vi "SIM BDF manager.vi"(1 "Simulation data":T1={"continuous integrator"=enum."RK 1 (Euler)", "initial time"=0.0, "final time"=6.0, "step size"=0.0, "proposed step size"=0.001, "max step size"=1e-06, "min step size"=0.0, "discrete time step"=0.0, "max step ratio"=3.0, "Diag Eval Stage"=enum."Major Substep", "Substep Index"=0, "Timestep Index"=10.0, "simulation time"=0.0, "current timestep base"=0.1, "proposed step time"=0.0, "absolute tolerance"=0.0, "relative tolerance"=0.0, "step accepted?"=FALSE, "step complete?"=FALSE, "Halt?"=FALSE, "reset integrator?"=FALSE, "machine epsilon"=1.0, "min float"=0.0, "error"={"status"=FALSE, "code"=0, "source"=""}, "Method Order"=0, "Finished Late [i-1]"=FALSE, "Discrete step?"=FALSE, "NaN and Inf check?"=FALSE, "Final Timestep Index"=0.0, "(maj+disc)or(init)?"=FALSE, "Full Solver Reset"=TRUE, "Execution Mode"=enum."Simulate to Completion", "check vector sizes?"=FALSE, "solver handles zc?"=FALSE, "Simulation Registry"={"Current Idx"=0, "Node Tags"=[], "Node Headers"=[], "Node Data"=[], "Cont State data"={"inputs"=[], "outputs"=[], "reset"=[], "lower limits"=[], "upper limits"=[], "limit types"=[], "reset types"=[], "initial conditions"=[], "reset I.C."=[], "limited?"=[], "State Names"=[]}, "DiscreteInfo"={"tick period (sec)"=0.0, "time (ticks)"=0, "fire?"=[], "registry"={"period (sec)"=[], "skew (sec)"=[], "period (tick)"=[], "skew (tick)"=[]}, "discrete \nblocks?"=FALSE, "steps per tick"=0.0, "steps to tick"=0.0, "discrete \ntick?"=FALSE}, "Disc State data"={"Disc States"=[], "State Names"=[]}, "Registry Error"={"Error Block ID"=0, "code"=0}, "ZC Indices"=[]}, "variable step solver?"=FALSE, "First Substep?"=FALSE, "Continuous States?"=FALSE} {"min float" format="%.1e"; "proposed step size" format="%.1e"; "proposed step time" format="%.1e"; "max step ratio" format="%.1e"; "min step size" format="%.1e"; "machine epsilon" format="%.1e"; "discrete time step" format="%.1e"; "max step size" format="%.1e"; "current timestep base" format="%.1e"; "final time" format="%.1e"; "simulation time" format="%.1e"; "relative tolerance" format="%.1e"; "absolute tolerance" format="%.1e"; "Substep Index" format="%.1e"; "step size" format="%.1e"; "initial time" format="%.1e"}) -> (0 "Simulation data out":T1={"continuous integrator"=enum."RK 1 (Euler)", "initial time"=0.0, "final time"=6.0, "step size"=0.0, "proposed step size"=0.001, "max step size"=1e-06, "min step size"=0.0, "discrete time step"=0.0, "max step ratio"=3.0, "Diag Eval Stage"=enum."Major Substep", "Substep Index"=0, "Timestep Index"=10.0, "simulation time"=0.0, "current timestep base"=0.1, "proposed step time"=0.0, "absolute tolerance"=0.0, "relative tolerance"=0.0, "step accepted?"=FALSE, "step complete?"=FALSE, "Halt?"=FALSE, "reset integrator?"=FALSE, "machine epsilon"=1.0, "min float"=0.0, "error"={"status"=FALSE, "code"=0, "source"=""}, "Method Order"=0, "Finished Late [i-1]"=FALSE, "Discrete step?"=FALSE, "NaN and Inf check?"=FALSE, "Final Timestep Index"=0.0, "(maj+disc)or(init)?"=FALSE, "Full Solver Reset"=TRUE, "Execution Mode"=enum."Simulate to Completion", "check vector sizes?"=FALSE, "solver handles zc?"=FALSE, "Simulation Registry"={"Current Idx"=0, "Node Tags"=[], "Node Headers"=[], "Node Data"=[], "Cont State data"={"inputs"=[], "outputs"=[], "reset"=[], "lower limits"=[], "upper limits"=[], "limit types"=[], "reset types"=[], "initial conditions"=[], "reset I.C."=[], "limited?"=[], "State Names"=[]}, "DiscreteInfo"={"tick period (sec)"=0.0, "time (ticks)"=0, "fire?"=[], "registry"={"period (sec)"=[], "skew (sec)"=[], "period (tick)"=[], "skew (tick)"=[]}, "discrete \nblocks?"=FALSE, "steps per tick"=0.0, "steps to tick"=0.0, "discrete \ntick?"=FALSE}, "Disc State data"={"Disc States"=[], "State Names"=[]}, "Registry Error"={"Error Block ID"=0, "code"=0}, "ZC Indices"=[]}, "variable step solver?"=FALSE, "First Substep?"=FALSE, "Continuous States?"=FALSE} {"min float" format="%.1e"; "proposed step size" format="%.1e"; "proposed step time" format="%.1e"; "max step ratio" format="%.1e"; "min step size" format="%.1e"; "machine epsilon" format="%.1e"; "discrete time step" format="%.1e"; "max step size" format="%.1e"; "current timestep base" format="%.1e"; "final time" format="%.1e"; "simulation time" format="%.1e"; "relative tolerance" format="%.1e"; "absolute tolerance" format="%.1e"; "Substep Index" format="%.1e"; "step size" format="%.1e"; "initial time" format="%.1e"})   [LabVIEW 2017]
uses:
  SIM simulation data.ctl
  SIM integration method.ctl
  SIM diagram eval stage.ctl
  SIMSCR Execution Mode.ctl
  SIM Simulation Registry.ctl
  SIM Registry Node Header.ctl
  SIM Registry Node Record.ctl
  SIM trigger type.ctl
  SIM solver state data.ctl
  SIM limit type.ctl
  SIM discrete data.ctl
  SIM Discrete state data.ctl
  SIM Simulation Registry Error.ctl
  SIM BDF stages.ctl
  SIM BDF data.ctl
  SIM Factored Matrix.ctl
panel:
  in  "Max Order":i32=5
  in  "max Newton iterations":i32=3
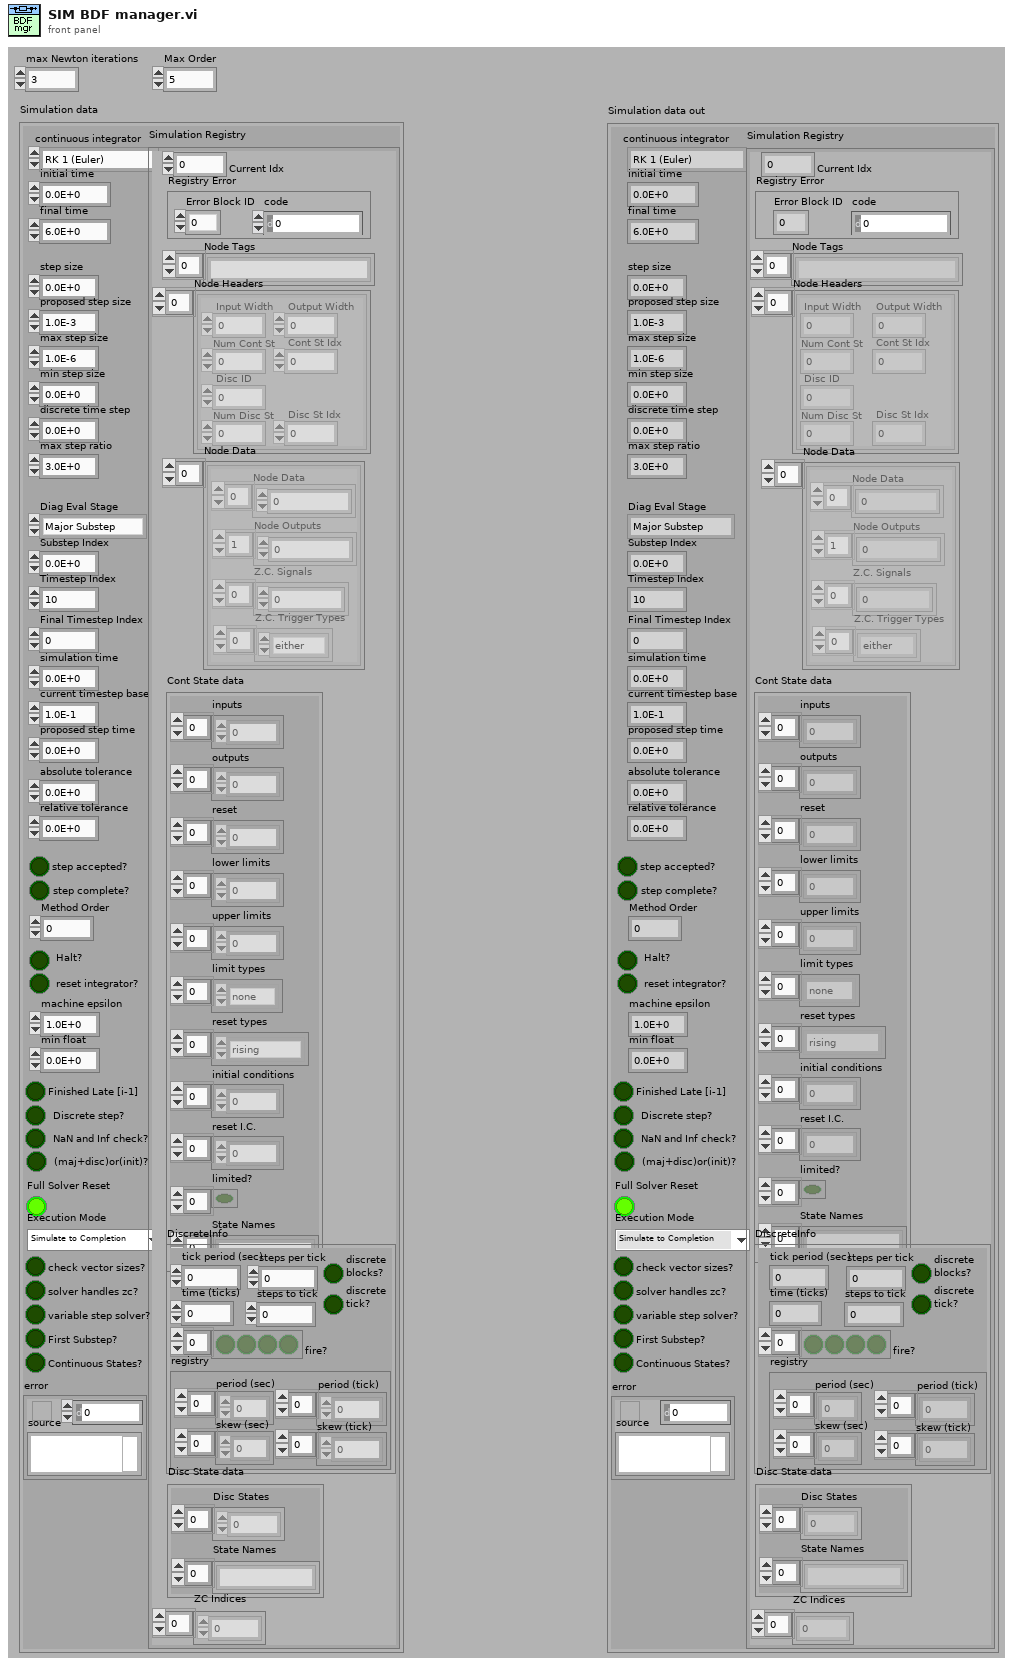
[diagram p1: front panel]
types:
  T1 = typedef "SIM simulation data.ctl" = cluster{"continuous integrator":T2, "initial time":dbl, "final time":dbl, "step size":dbl, "proposed step size":dbl, "max step size":dbl, "min step size":dbl, "discrete time step":dbl, "max step ratio":dbl, "Diag Eval Stage":T3, "Substep Index":i32, "Timestep Index":dbl, "simulation time":dbl, "current timestep base":dbl, "proposed step time":dbl, "absolute tolerance":dbl, "relative tolerance":dbl, "step accepted?":bool, "step complete?":bool, "Halt?":bool, "reset integrator?":bool, "machine epsilon":dbl, "min float":dbl, "error":errorcluster, "Method Order":u32, "Finished Late [i-1]":bool, "Discrete step?":bool, "NaN and Inf check?":bool, "Final Timestep Index":dbl, "(maj+disc)or(init)?":bool, "Full Solver Reset":bool, "Execution Mode":T4, "check vector sizes?":bool, "solver handles zc?":bool, "Simulation Registry":T5, "variable step solver?":bool, "First Substep?":bool, "Continuous States?":bool}
  T2 = typedef "SIM integration method.ctl" = enum16{"RK 1 (Euler)", "Linearizer", "State Query", "Trim Eval", "Adams", "RK 3", "RK 4", "RK 45", "BDF", "RK 2", "RK 23", "Rosenbrock", "Discrete States Only"}
  T3 = typedef "SIM diagram eval stage.ctl" = enum16{"Init", "Minor Substep", "Major Substep", "Final"}
  T4 = typedef "SIMSCR Execution Mode.ctl" = enum16{"Simulate to Completion", "Single Time-Step Simulation (Fixed Step Only)"}
  T5 = typedef "SIM Simulation Registry.ctl" = cluster{"Current Idx":i32, "Node Tags":string[], "Node Headers":T6[], "Node Data":T7[], "Cont State data":T9, "DiscreteInfo":T11, "Disc State data":T12, "Registry Error":T13, "ZC Indices":i32[]}
  T6 = typedef "SIM Registry Node Header.ctl" = cluster{"Input Width":i32, "Disc ID":i32, "Num Cont St":i32, "Cont St Idx":i32, "Num Disc St":i32, "Disc St Idx":i32, "Output Width":i32}
  T7 = typedef "SIM Registry Node Record.ctl" = cluster{"Node Data":dbl[], "Node Outputs":dbl[], "Z.C. Signals":dbl[], "Z.C. Trigger Types":T8[]}
  T8 = typedef "SIM trigger type.ctl" = enum16{"rising", "falling", "either", "none"}
  T9 = typedef "SIM solver state data.ctl" = cluster{"inputs":dbl[], "outputs":dbl[], "reset":dbl[], "lower limits":dbl[], "upper limits":dbl[], "limit types":T10[], "reset types":T8[], "initial conditions":dbl[], "reset I.C.":dbl[], "limited?":bool[], "State Names":string[]}
  T10 = typedef "SIM limit type.ctl" = enum16{"upper", "lower", "both", "none"}
  T11 = typedef "SIM discrete data.ctl" = cluster{"tick period (sec)":dbl, "time (ticks)":i32, "fire?":bool[], "registry":cluster{"period (sec)":dbl[], "skew (sec)":dbl[], "period (tick)":i32[], "skew (tick)":i32[]}, "discrete \nblocks?":bool, "steps per tick":dbl, "steps to tick":dbl, "discrete \ntick?":bool}
  T12 = typedef "SIM Discrete state data.ctl" = cluster{"Disc States":dbl[], "State Names":string[]}
  T13 = typedef "SIM Simulation Registry Error.ctl" = cluster{"Error Block ID":i32, "code":i32}
  T14 = typedef "SIM BDF stages.ctl" = enum16{"Init", "Initial Guess", "Compute Jacobian", "Newton Iteration", "Eval Error", "Choose StepSize", "Reset BDFs"}
  T15 = typedef "SIM BDF data.ctl" = cluster{"BDFs":dbl[][], "init. guess (y*)":dbl[], "p'(y*)":dbl[], "Factored jacobian":T16, "zero array":dbl[], "reinit Jac.":bool, "BDF stage":T14, "steps this jac":i32, "time index this jac":i32, "Number of jac evals":i32, "del_k":dbl[], "Current Order":i32, "Max Order":i32, "Steps This Order":i32, "Max Err Order":i32}
  T16 = typedef "SIM Factored Matrix.ctl" = cluster{"L":dbl[][], "U":dbl[][], "P":i32[][]}
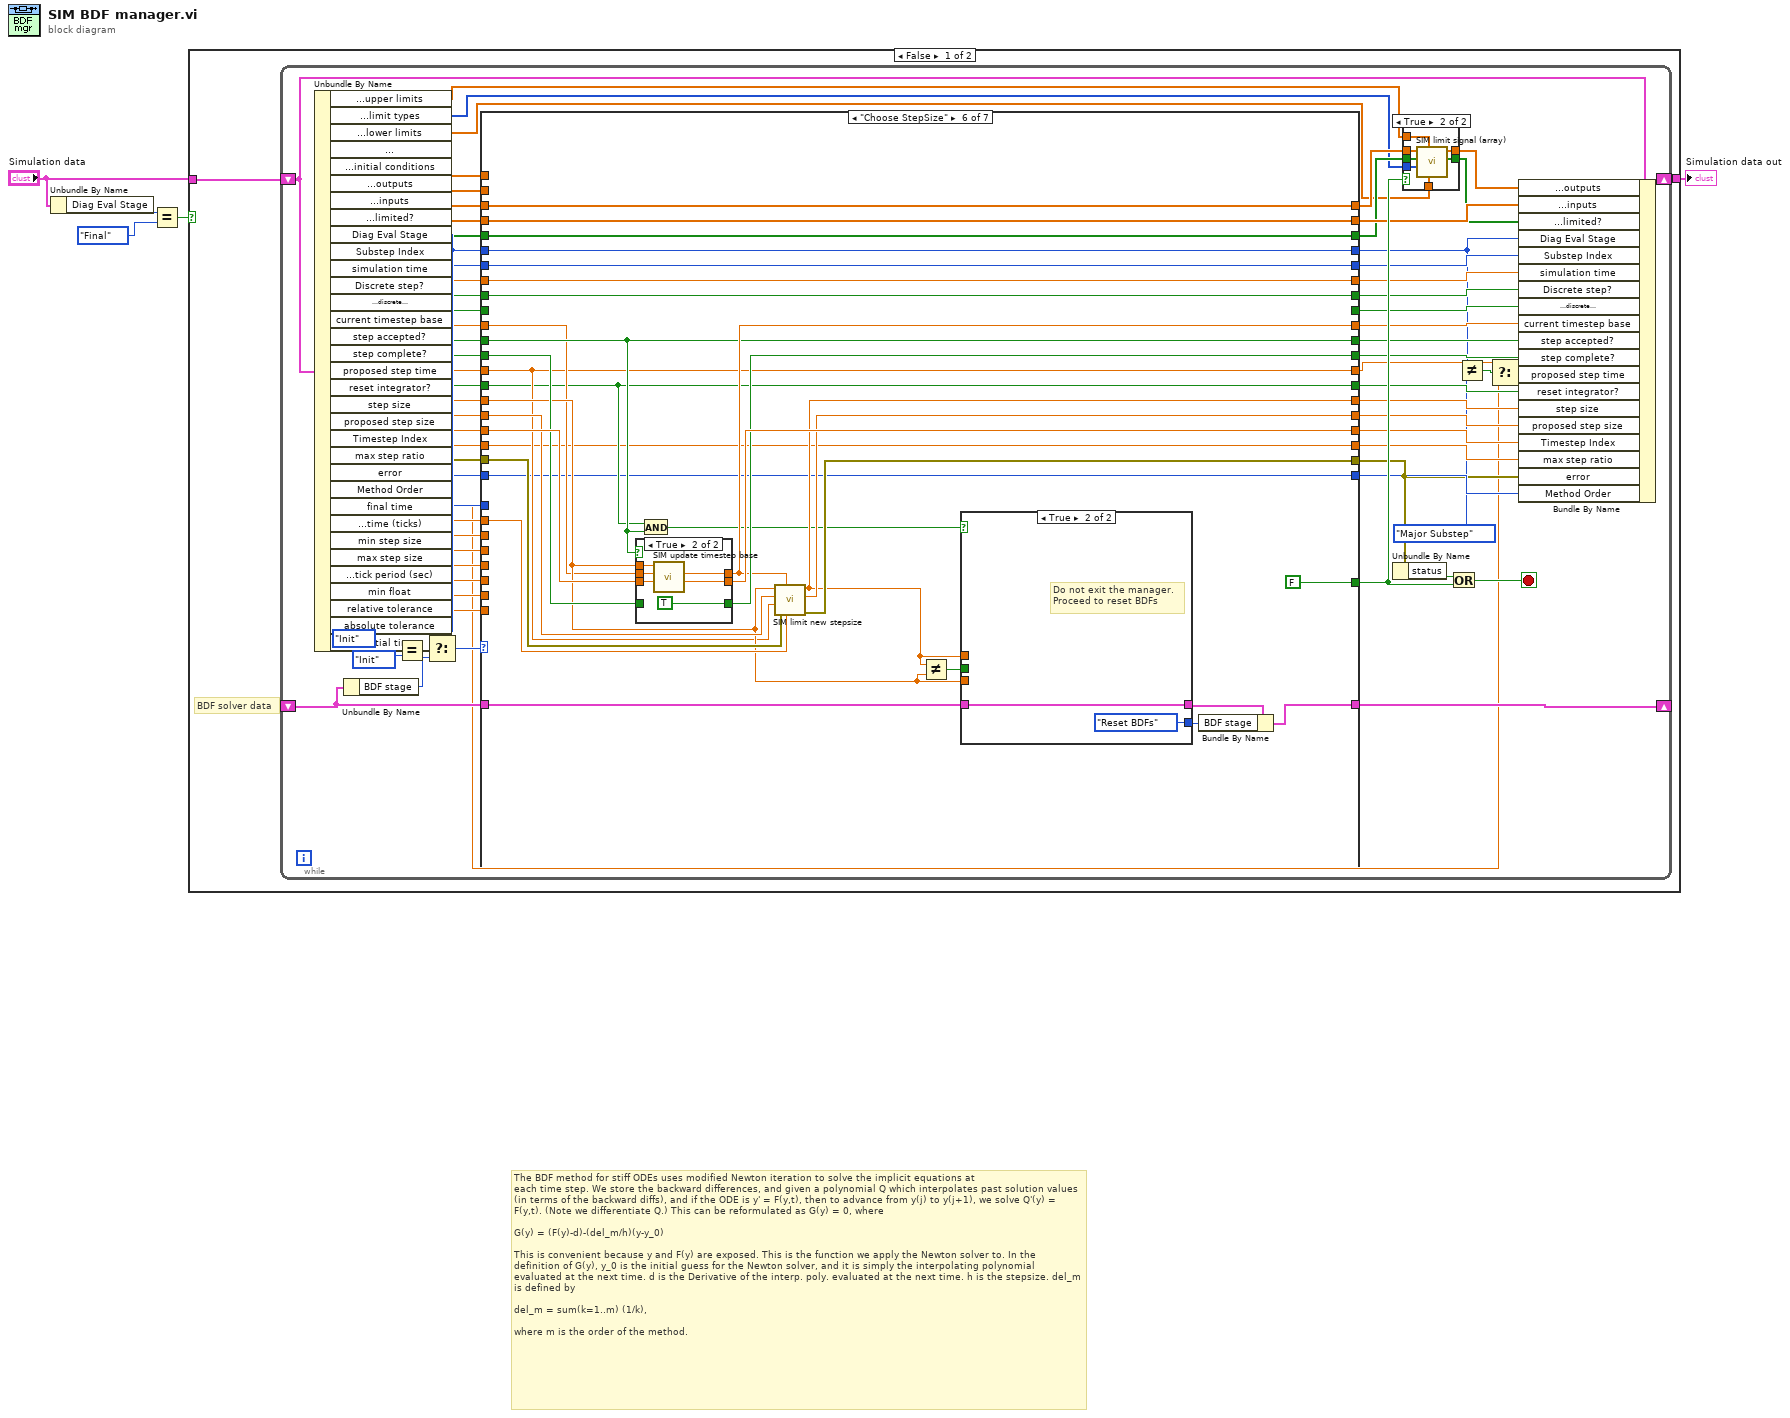
[diagram p0: block diagram]
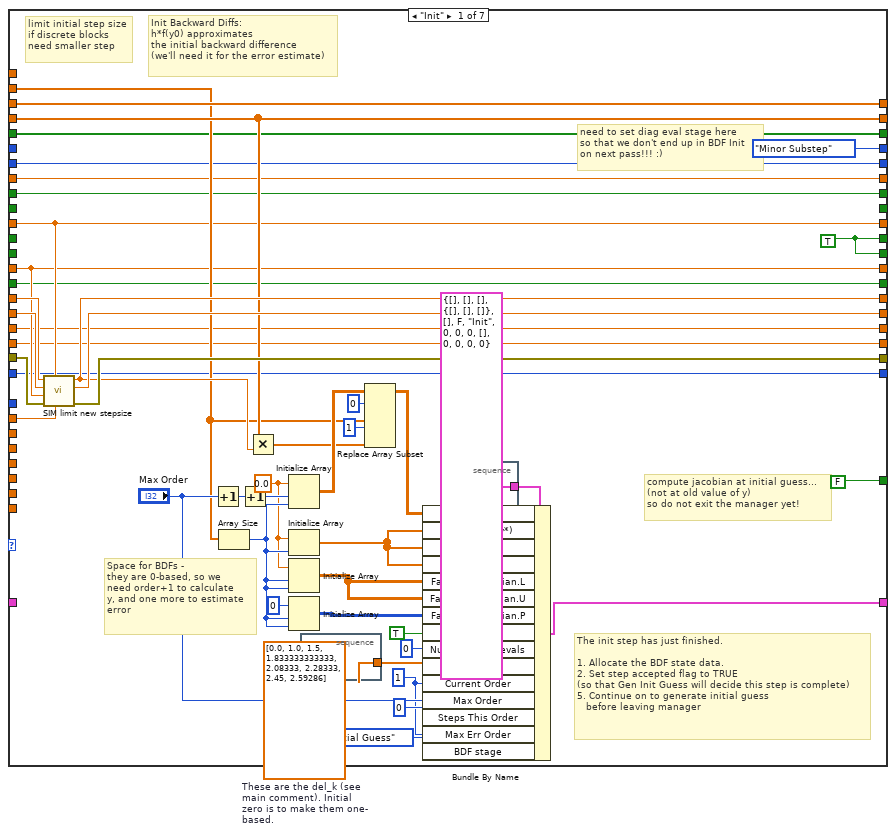
[diagram p3: hidden frame]
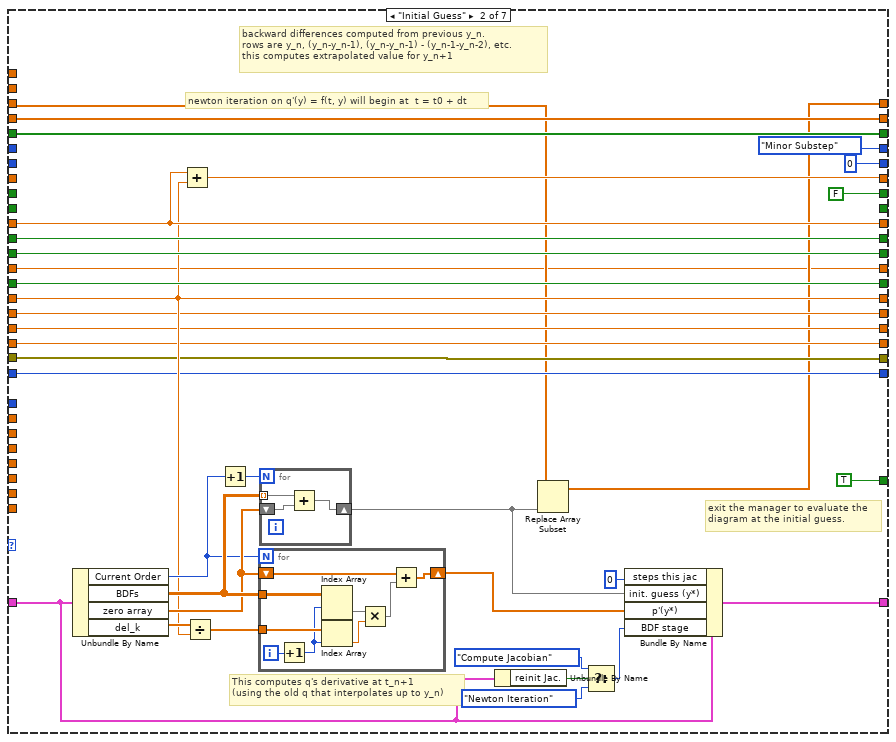
[diagram p4: hidden frame]
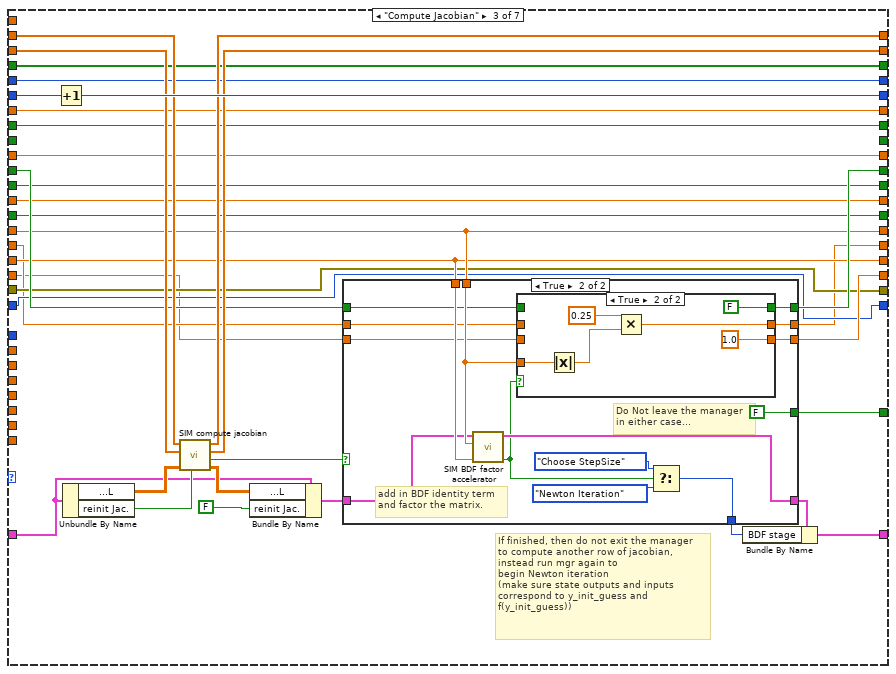
[diagram p5: hidden frame]
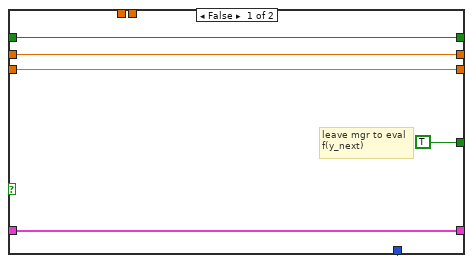
[diagram p6: hidden frame]
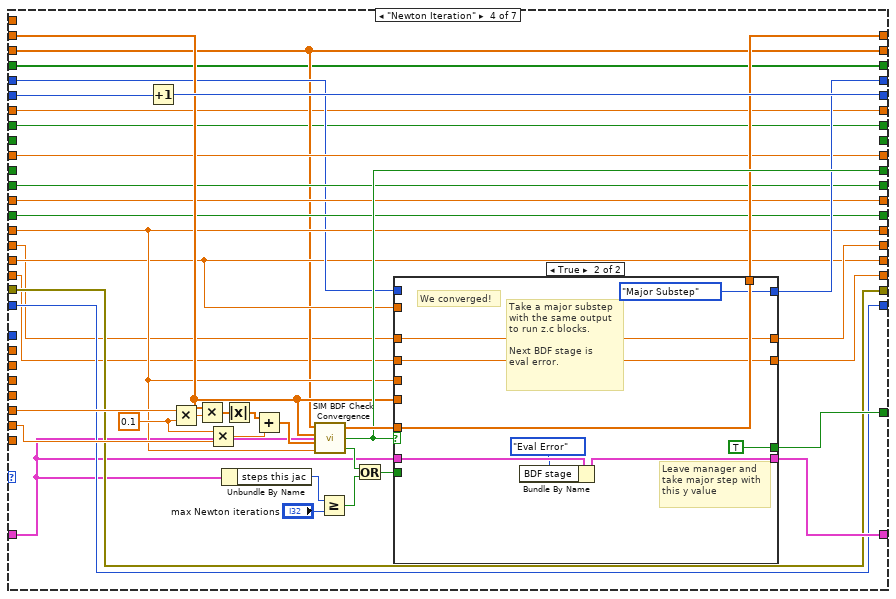
[diagram p8: hidden frame]
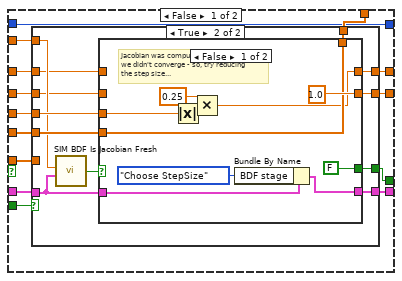
[diagram p9: hidden frame]
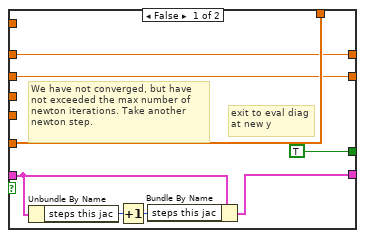
[diagram p10: hidden frame]
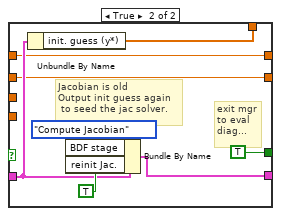
[diagram p11: hidden frame]
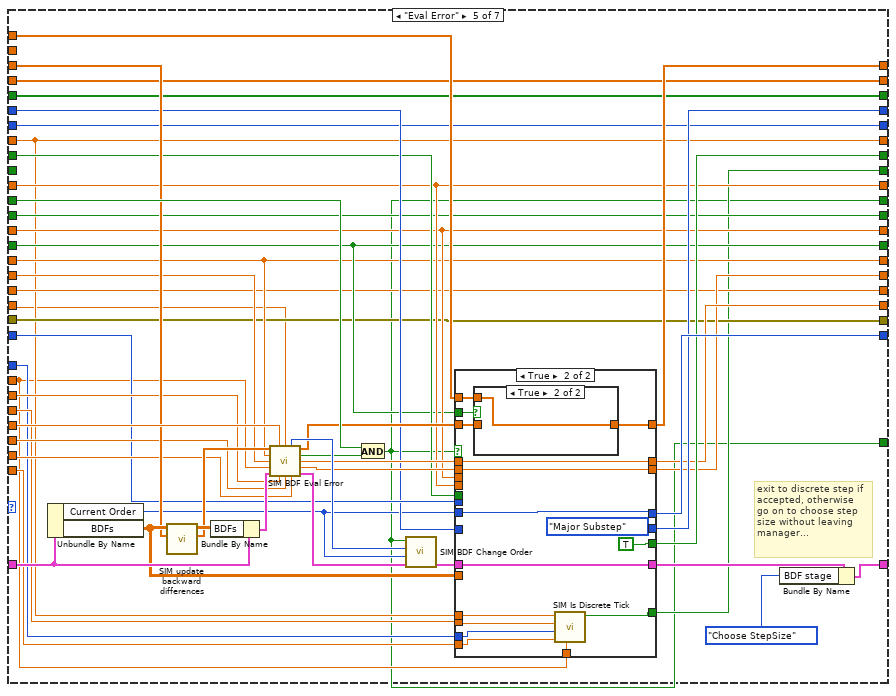
[diagram p12: hidden frame]
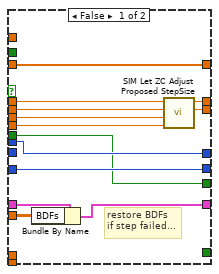
[diagram p13: hidden frame]
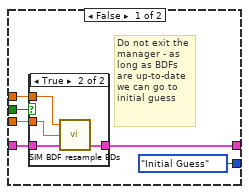
[diagram p15: hidden frame]
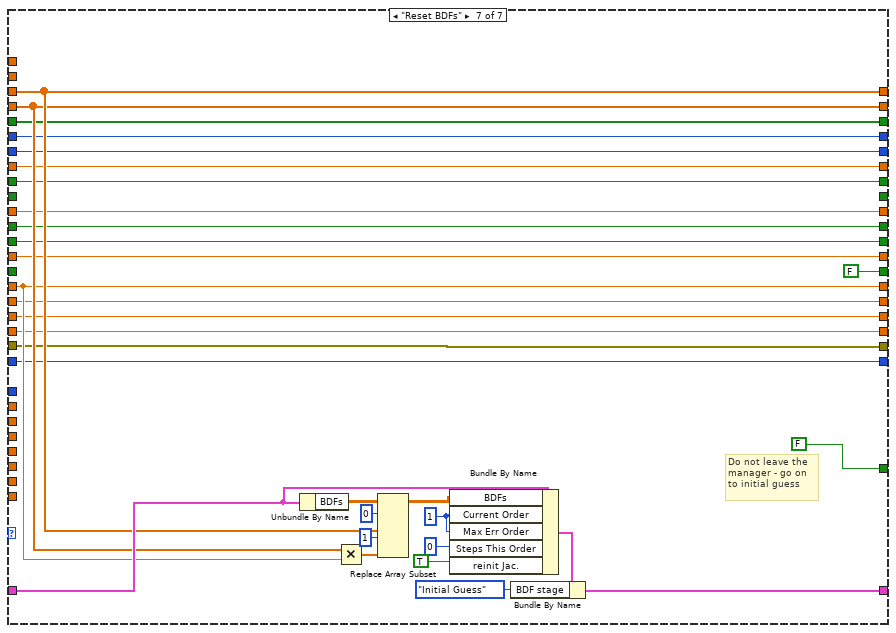
[diagram p18: hidden frame]
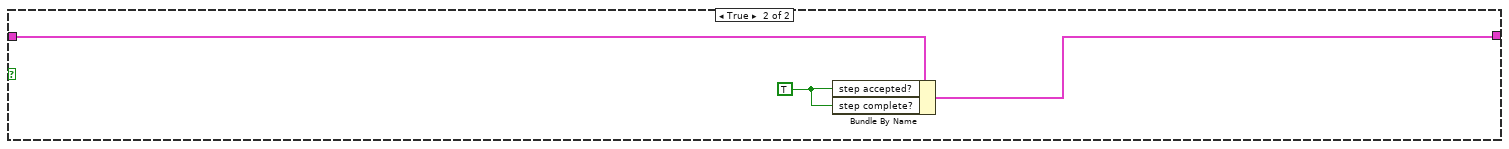
[diagram p19: hidden frame]
diagram:
  # "The BDF method for stiff ODEs uses modified Newton iteration to solve the implicit equations at\neach time step. We store the backward differences, and given a polynomial Q which interpolates past solution values (in terms of the backward diffs), and if the ODE is y' = F(y,t), then to advance from y(j) to y(j+1), we solve Q'(y) = F(y,t). (Note we differentiate Q.) This can be reformulated as G(y) = 0, where \n\nG(y) = (F(y)-d)-(del_m/h)(y-y_0)\n\nThis is convenient because y and F(y) are exposed. This is the function we apply the Newton solver to. In the definition of G(y), y_0 is the initial guess for the Newton solver, and it is simply the interpolating polynomial evaluated at the next time. d is the Derivative of the interp. poly. evaluated at the next time. h is the stepsize. del_m is defined by\n\ndel_m = sum(k=1..m) (1/k),\n\nwhere m is the order of the method."
  n1 = Unbundle By Name("Simulation data") -> ("Diag Eval Stage"=w3:T3)
  n2 = Equal?(x=w3, y=SIM_diagram_eval_stage."Final") -> (x = y?=w1:bool)
  n3 = case shown="False" w1 {
    tunnel: [w7 w513] -> w5
    tunnel: "Simulation data" -> [w6 w512]
    frame False {
      # "BDF solver data"
      n4 = while {
        shift-right: [w37] -> w7
        shift-left: w6 -> [w17]
        shift-right: [w70] -> _
        shift-left: _ -> [w73]
        stop <- w74 stop-if-true
        n5 = Unbundle By Name(w17) -> ("Simulation Registry.Cont State data.upper limits"=w20:dbl[], "Simulation Registry.Cont State data.limit types"=w18:T10[], "Simulation Registry.Cont State data.lower limits"=w19:dbl[], "Simulation Registry.Cont State data.reset I.C."=w29:dbl[], "Simulation Registry.Cont State data.initial conditions"=w32:dbl[], "Simulation Registry.Cont State data.outputs"=w41:dbl[], "Simulation Registry.Cont State data.inputs"=w40:dbl[], "Simulation Registry.Cont State data.limited?"=w34:bool[], "Diag Eval Stage"=w67:T3, "Substep Index"=w66:i32, "simulation time"=w64:dbl, "Discrete step?"=w62:bool, "Simulation Registry.DiscreteInfo.discrete \ntick?"=w60:bool, "current timestep base"=w58:dbl, "step accepted?"=w56:bool, "step complete?"=w54:bool, "proposed step time"=w52:dbl, "reset integrator?"=w51:bool, "step size"=w49:dbl, "proposed step size"=w47:dbl, "Timestep Index"=w45:dbl, "max step ratio"=w43:dbl, "error"=w27:errorcluster, "Method Order"=w26:u32, "final time"=w10:dbl, "Simulation Registry.DiscreteInfo.time (ticks)"=w16:i32, "min step size"=w33:dbl, "max step size"=w30:dbl, "Simulation Registry.DiscreteInfo.tick period (sec)"=w38:dbl, "min float"=w31:dbl, "relative tolerance"=w36:dbl, "absolute tolerance"=w35:dbl, "initial time"=w15:dbl)
        n6 = Unbundle By Name(w73) -> ("BDF stage"=w72:T14)
        n7 = Equal?(x=w67, y=SIM_diagram_eval_stage."Init") -> (x = y?=w69:bool)
        n8 = Select(t=SIM_BDF_stages."Init" ("Enum"), s=w69, f=w72) -> (s? t:f=w11:T14)
        n9 = case shown="\"Choose StepSize\"" w11 {
          tunnel: [FALSE TRUE w204 w283 w345 FALSE FALSE ("finished?")] -> w68
          tunnel: [w111 w167 w206 w284 w390 w455 w508] -> w70
          tunnel: w73 -> [_ w163 w210 w249 w394 w457 w499]
          tunnel: [SIM_diagram_eval_stage."Minor Substep" ("Diag Eval Stage") SIM_diagram_eval_stage."Minor Substep" ("Diagram Eval Stage") w197 w264 w374 w439 w495] -> w12
          tunnel: w67 -> [_ _ w197 w255 w367 w439 w495]
          tunnel: [w94 0 ("Substep Index") w202 w267 w362 w438 w494] -> w65
          tunnel: w66 -> [w94 _ w203 w268 w362 w438 w494]
          tunnel: w64 -> [w93 _ w193 w246 w352 w437 w493]
          tunnel: [w93 w149 w193 w246 w352 w437 w493] -> w63
          tunnel: [w92 FALSE ("Discrete step?") w192 w245 w373 w436 w492] -> w61
          tunnel: w62 -> [w92 _ w192 w245 w366 w436 w492]
          tunnel: w60 -> [_ _ _ _ _ _ _]
          tunnel: [_ _ _ _ w353 _ _] -> w59
          tunnel: [w91 w146 w191 w260 w361 w442 w491] -> w57
          tunnel: w58 -> [w91 w146 w191 w260 w361 w434 w491]
          tunnel: [w100 w145 w195 w266 w345 w435 w490] -> w55
          tunnel: w56 -> [_ w145 w194 _ w389 w435 w490]
          tunnel: [w100 w144 w190 w259 w360 w450 w489] -> w53
          tunnel: w54 -> [_ w144 w190 w259 w360 w451 w489]
          tunnel: [w90 w133 w183 w258 w359 w433 w488] -> w9
          tunnel: w52 -> [w90 w133 w183 w258 w359 w433 w488]
          tunnel: [w89 w143 w189 w257 w358 w432 FALSE ("reset integrator?")] -> w50
          tunnel: w51 -> [w89 w143 w189 w257 w358 w432 _]
          tunnel: [w101 w142 w188 w256 w357 w444 w487] -> w48
          tunnel: w49 -> [w107 w142 w188 w256 w357 w443 w487]
          tunnel: [w103 w141 w182 w262 w371 w446 w486] -> w46
          tunnel: w47 -> [w106 w141 w181 w248 w383 w449 w486]
          tunnel: [w88 w140 w187 w254 w356 w452 w485] -> w44
          tunnel: w45 -> [w88 w140 w187 w254 w356 w453 w485]
          tunnel: [w87 w139 w196 w263 w372 w430 w484] -> w42
          tunnel: w43 -> [w87 w139 w180 w247 w351 w430 w484]
          tunnel: w41 -> [w98 w135 w201 w261 w385 w429 w498]
          tunnel: w40 -> [w97 w147 w200 w253 w364 w441 w497]
          tunnel: [w98 w134 w199 w265 w365 w429 w498] -> w24
          tunnel: [w97 w147 w198 w253 w364 w441 w497] -> w39
          tunnel: w38 -> [_ _ _ _ w354 _ _]
          tunnel: w36 -> [_ _ _ w270 w381 _ _]
          tunnel: w35 -> [_ _ _ w269 w380 _ _]
          tunnel: w34 -> [w95 w148 w184 w252 w363 w440 w496]
          tunnel: w27 -> [w105 w138 w186 w251 w355 w448 w483]
          tunnel: w33 -> [w104 _ _ _ w347 w447 _]
          tunnel: [w102 w138 w186 w251 w355 w445 w483] -> w25
          tunnel: w32 -> [w96 _ _ _ _ _ _]
          tunnel: [w95 w148 w184 w252 w363 w440 w496] -> w21
          tunnel: w31 -> [_ _ _ _ w386 _ _]
          tunnel: w30 -> [_ _ _ _ w382 _ _]
          tunnel: w29 -> [_ _ _ _ w377 _ _]
          tunnel: [w86 w137 w185 w250 w375 w431 w482] -> w28
          tunnel: w26 -> [w86 w137 w185 w250 w368 w431 w482]
          tunnel: w16 -> [_ _ _ _ w350 _ _]
          tunnel: w15 -> [_ _ _ _ w348 _ _]
          frame "Init" {
            w100 = TRUE ("step complete?")
            w108 = 1 ("Current Order")
            w122 = 0.0
            # "limit initial step size\nif discrete blocks\nneed smaller step"
            # "need to set diag eval stage here\nso that we don't end up in BDF Init\non next pass!!! :)"
            # "Init Backward Diffs:\nh*f(y0) approximates\nthe initial backward difference\n(we'll need it for the error estimate)"
            # "Space for BDFs - \nthey are 0-based, so we\nneed order+1 to calculate\ny, and one more to estimate\nerror"
            # "compute jacobian at initial guess...\n(not at old value of y)\nso do not exit the manager yet!"
            # "The init step has just finished.\n\n1. Allocate the BDF state data.\n2. Set step accepted flag to TRUE\n(so that Gen Init Guess will decide this step is complete)\n5. Continue on to generate initial guess\n   before leaving manager"
            n10 = call "SIM limit new stepsize.vi"("min step size"=w104, "current timestep base"=w91, "error"=w105, "proposed step time"=w90, "proposed step size"=w106, "step size"=w107) -> ("error out"=w102:errorcluster, "proposed step size"=w103:dbl, "step size"=w101:dbl)  [unwired: 3 out]
            n11 = Increment(x="Max Order") -> (x+1=w115:i32)
            n12 = Array Size(array=w96) -> (size(s)=w123:i32)
            n13 = Increment(x=w115) -> (x+1=w128:i32)
            n14 = Multiply(x=w97, y=w101) -> (x*y=w114:dbl[])
            n15 = Initialize Array(w122, w128, w123) -> (w120:dbl[][])
            n16 = Initialize Array(w122, w123) -> (w119:dbl[])
            n17 = Initialize Array(w122, w123, w123) -> (w126:dbl[][])
            n18 = Initialize Array(0, w123, w123) -> (w125:i32[][])
            n19 = stacked-sequence {
              tunnel: [w132] -> w116
              frame #0 {
                w132 = dbl[] [0.0, 1.0, 1.5, 1.833333333333, 2.08333, 2.28333, 2.45, 2.59286]  # These are the del_k (see main comment). Initial zero is to make them one- based.
              }
            }
            n20 = Replace Array Subset(array=w120, new element #1=w96, index (row) #1=0, new element #2=w114, index (row) #2=1 ("index (row)")) -> (w127:dbl[][])  [unwired: 2 in]
            n21 = stacked-sequence {
              tunnel: [T15 {"BDFs"=[], "init. guess (y*)"=[], "p'(y*)"=[], "Factored jacobian"={"L"=[], "U"=[], "P"=[]}, "zero array"=[], "reinit Jac."=FALSE, "BDF stage"=enum."Init", "steps this jac"=0, "time index this jac"=0, "Number of jac evals"=0, "del_k"=[], "Current Order"=0, "Max Order"=0, "Steps This Order"=0, "Max Err Order"=0} ("BDF data")] -> w118
              frame #0 {
              }
            }
            n22 = Bundle By Name(cluster=w118, "BDFs"=w127, "init. guess (y*)"=w119, "p'(y*)"=w119, "zero array"=w119, "Factored jacobian.L"=w126, "Factored jacobian.U"=w126, "Factored jacobian.P"=w125, "reinit Jac."=TRUE, "Number of jac evals"=0, "del_k"=w116, "Current Order"=w108, "Max Order"="Max Order", "Steps This Order"=0, "Max Err Order"=w108, "BDF stage"=SIM_BDF_stages."Initial Guess" ("Enum")) -> (w111:T15)
          }
          frame "Initial Guess" {
            # "newton iteration on q'(y) = f(t, y) will begin at  t = t0 + dt"
            # "This computes q's derivative at t_n+1\n(using the old q that interpolates up to y_n)"
            # "backward differences computed from previous y_n.\nrows are y_n, (y_n-y_n-1), (y_n-y_n-1) - (y_n-1-y_n-2), etc.\nthis computes extrapolated value for y_n+1"
            # "exit the manager to evaluate the \ndiagram at the initial guess."
            n23 = Unbundle By Name(w163) -> ("Current Order"=w153:i32, "BDFs"=w165:dbl[][], "zero array"=w164:dbl[], "del_k"=w154:dbl[])
            n24 = Add(x=w146, y=w142) -> (x+y=w149:dbl)
            n25 = Divide(x=w154, y=w142) -> (x/y=w156:dbl[])
            n26 = Increment(x=w153) -> (x+1=w157:i32)
            n27 = for {
              N: w153 -> [_]
              shift-right: [w173] -> w155
              shift-left: w164 -> [w174]
              tunnel: w165 -> [w168]
              tunnel: w156 -> [w176]
              i -> [w170]
              n28 = Increment(x=w170) -> (x+1=w169:i32)
              n29 = Index Array(array=w168, index (row)=w169) -> (element=w171:dbl[])  [unwired: 1 in]
              n30 = Index Array(array=w176, index=w169) -> (element=w172:dbl)
              n31 = Multiply(x=w171, y=w172) -> (x*y=w175:dbl[])
              n32 = Add(x=w174, y=w175) -> (x+y=w173:dbl[])
            }
            n33 = for {
              N: w157 -> [_]
              shift-right: [w178] -> w136
              shift-left: w164 -> [w179]
              tunnel: w165 -> [w177] mode=indexing
              n34 = Add(x=w177, y=w179) -> (x+y=w178:dbl[])
            }
            n35 = Unbundle By Name(w163) -> ("reinit Jac."=w162:bool)
            n36 = Replace Array Subset(array=w135, new element=w136) -> (w134:dbl[])  [unwired: 1 in]
            n37 = Select(t=SIM_BDF_stages."Compute Jacobian" ("BDF stage"), s=w162, f=SIM_BDF_stages."Newton Iteration" ("BDF stage")) -> (s? t:f=w159:T14)
            n38 = Bundle By Name(cluster=w163, "steps this jac"=0, "init. guess (y*)"=w136, "p'(y*)"=w155, "BDF stage"=w159) -> (w167:T15)
          }
          frame "Compute Jacobian" {
            # "If finished, then do not exit the manager\nto compute another row of jacobian,\ninstead run mgr again to \nbegin Newton iteration\n(make sure state outputs and inputs\ncorrespond to y_init_guess and\nf(y_init_guess))"
            n39 = Increment(x=w203) -> (x+1=w202:i32)
            n40 = Unbundle By Name(w210) -> ("Factored jacobian.L"=w214:dbl[][], "reinit Jac."=w213:bool)
            n41 = call "SIM compute jacobian.vi"("reset?"=w213, "Current jacobian"=w214, "F(y)"=w200, "y current"=w201) -> ("Current jacobian out"=w212:dbl[][], "finished?"=w209:bool, "F(y_0)"=w198:dbl[], "y next"=w199:dbl[])  [unwired: 2 in, 2 out]
            n42 = Bundle By Name(cluster=w210, "Factored jacobian.L"=w212, "reinit Jac."=FALSE ("need jac module re-init")) -> (w208:T15)
            n43 = case shown="True" w209 {
              tunnel: w208 -> [w219 w227]
              tunnel: [w219 w234] -> w207
              tunnel: [SIM_BDF_stages."Compute Jacobian" ("Enum") w230] -> w205
              tunnel: [TRUE FALSE] -> w204
              tunnel: w188 -> [_ w228]
              tunnel: w187 -> [_ w229]
              tunnel: [w216 w226] -> w182
              tunnel: [w217 w225] -> w196
              tunnel: [w215 w224] -> w195
              tunnel: w180 -> [w217 w222]
              tunnel: w181 -> [w216 w221]
              tunnel: w194 -> [w215 w223]
              frame False {
                # "leave mgr to eval\nf(y_next)"
              }
              frame True {
                # "Do Not leave the manager\nin either case..."
                # "add in BDF identity term\nand factor the matrix."
                n44 = call "SIM BDF factor accelerator.vi"("current timestep index"=w229, "step size"=w228, "BDF data"=w227) -> ("error"=w233:bool, "BDF data out"=w234:T15)  [unwired: 1 in, 6 out]
                n45 = case shown="True" w233 {
                  tunnel: w228 -> [_ w242]
                  tunnel: [w236 w241] -> w226
                  tunnel: [w237 1.0 ("max step ratio")] -> w225
                  tunnel: [w238 FALSE ("step accepted?")] -> w224
                  tunnel: w223 -> [w238 _]
                  tunnel: w222 -> [w237 _]
                  tunnel: w221 -> [w236 _]
                  frame False {
                  }
                  frame True {
                    n46 = Absolute Value(x=w242) -> (abs(x)=w243:dbl)
                    n47 = Multiply(x=0.25, y=w243) -> (x*y=w241:dbl)
                  }
                }
                n48 = Select(t=SIM_BDF_stages."Choose StepSize", s=w233, f=SIM_BDF_stages."Newton Iteration" ("Enum")) -> (s? t:f=w230:T14)
              }
            }
            n49 = Bundle By Name(cluster=w207, "BDF stage"=w205) -> (w206:T15)
          }
          frame "Newton Iteration" {
            w276 = 0.1 ("y")
            n50 = Increment(x=w268) -> (x+1=w267:i32)
            n51 = Multiply(x=w270, y=w276) -> (x*y=w278:dbl)
            n52 = Multiply(x=w261, y=w278) -> (x*y=w281:dbl[])
            n53 = Multiply(x=w276, y=w269) -> (x*y=w277:dbl)
            n54 = Unbundle By Name(w249) -> ("steps this jac"=w274:i32)
            n55 = Absolute Value(x=w281) -> (abs(x)=w280:dbl[])
            n56 = Add(x=w280, y=w277) -> (x+y=w282:dbl[])
            n57 = call "SIM BDF Check Convergence.vi"("f(y)"=w253, "y"=w261, "err tolerance"=w282, "step size"=w256, "BDF data"=w249) -> ("y next"=w279:dbl[], "converged?"=w266:bool, "Newton Error?"=w271:bool)
            n58 = Greater Or Equal?(x=w274, y="max Newton iterations") -> (x >= y?=w272:bool)
            n59 = Or(x=w271, y=w272) -> (x .or. y?=w273:bool)
            n60 = case shown="True" w266 {
              tunnel: w279 -> [w298 w340]
              tunnel: w249 -> [w297 w344]
              tunnel: [w296 w341] -> w284
              tunnel: [w295 TRUE ("finished?")] -> w283
              tunnel: w273 -> [w294 _]
              tunnel: [w293 w340] -> w265
              tunnel: [w285 SIM_diagram_eval_stage."Major Substep" ("Diagram Eval Stage")] -> w264
              tunnel: [w292 w338] -> w263
              tunnel: [w291 w337] -> w262
              tunnel: w256 -> [w290 _]
              tunnel: w261 -> [w289 _]
              tunnel: w254 -> [w288 _]
              tunnel: w248 -> [w287 w337]
              tunnel: w247 -> [w286 w338]
              tunnel: w255 -> [w285 _]
              frame False {
                n61 = case shown="True" w294 {
                  tunnel: w298 -> [w301 _]
                  tunnel: w297 -> [w303 w315]
                  tunnel: [w305 w316] -> w296
                  tunnel: [TRUE w317] -> w295
                  tunnel: [w301 w311] -> w293
                  tunnel: [w299 w314] -> w292
                  tunnel: [w300 w313] -> w291
                  tunnel: w290 -> [_ w312]
                  tunnel: w289 -> [_ w310]
                  tunnel: w288 -> [_ w309]
                  tunnel: w287 -> [w300 w308]
                  tunnel: w286 -> [w299 w307]
                  frame False {
                    # "exit to eval diag\nat new y"
                    # "We have not converged, but have\nnot exceeded the max number of \nnewton iterations. Take another\nnewton step."
                    n62 = Unbundle By Name(w303) -> ("steps this jac"=w302:i32)
                    n63 = Increment(x=w302) -> (x+1=w306:i32)
                    n64 = Bundle By Name(cluster=w303, "steps this jac"=w306) -> (w305:T15)
                  }
                  frame True {
                    n65 = call "SIM BDF Is Jacobian Fresh.vi"("BDF data out"=w315, "Timestep Index"=w309) -> ("Old Jacobian?"=w318:bool)  [unwired: 4 out]
                    n66 = case shown="False" w318 {
                      tunnel: w315 -> [w325 w332]
                      tunnel: [FALSE TRUE] -> w317
                      tunnel: [w326 w333] -> w316
                      tunnel: [1.0 ("max step ratio") w329] -> w314
                      tunnel: [w319 w330] -> w313
                      tunnel: w312 -> [w321 _]
                      tunnel: [w320 w331] -> w311
                      tunnel: w310 -> [w320 _]
                      tunnel: w308 -> [_ w330]
                      tunnel: w307 -> [_ w329]
                      frame False {
                        # "Jacobian was computed at this step, and\nwe didn't converge - so, try reducing\nthe step size..."
                        n67 = Absolute Value(x=w321) -> (abs(x)=w323:dbl)
                        n68 = Multiply(x=0.25, y=w323) -> (x*y=w319:dbl)
                        n69 = Bundle By Name(cluster=w325, "BDF stage"=SIM_BDF_stages."Choose StepSize") -> (w326:T15)
                      }
                      frame True {
                        # "exit mgr\nto eval\ndiag..."
                        # "Jacobian is old\nOutput init guess again\n to seed the jac solver."
                        n70 = Unbundle By Name(w332) -> ("init. guess (y*)"=w331:dbl[])
                        n71 = Bundle By Name(cluster=w332, "BDF stage"=SIM_BDF_stages."Compute Jacobian", "reinit Jac."=TRUE) -> (w333:T15)
                      }
                    }
                  }
                }
              }
              frame True {
                # "Leave manager and\ntake major step with\nthis y value"
                # "We converged!"
                # "Take a major substep\nwith the same output\nto run z.c blocks.\n\nNext BDF stage is \neval error."
                n72 = Bundle By Name(cluster=w344, "BDF stage"=SIM_BDF_stages."Eval Error") -> (w341:T15)
              }
            }
          }
          frame "Eval Error" {
            # "exit to discrete step if\naccepted, otherwise\ngo on to choose step \nsize without leaving\nmanager..."
            n73 = Unbundle By Name(w394) -> ("Current Order"=w349:i32, "BDFs"=w393:dbl[][])
            n74 = call "SIM update backward differences.vi"("New y"=w385, "Backward differences"=w393) -> ("New y out"=w384:dbl[], "New Backward differences"=w395:dbl[][])  [unwired: 8 out]
            n75 = Bundle By Name(cluster=w394, "BDFs"=w395) -> (w388:T15)
            n76 = call "SIM BDF Eval Error.vi"("outputs"=w384, "min float"=w386, "max step ratio"=w351, "step size"=w357, "proposed step size"=w383, "min step size"=w347, "BDF data"=w388, "max step size"=w382, "relative tolerance"=w381, "absolute tolerance"=w380) -> ("proposed new order out"=w379:i32, "outputs out"=w376:dbl[], "step accepted? out"=w378:bool, "proposed max step ratio out"=w370:dbl, "proposed step size out"=w369:dbl, "BDF data out"=w387:T15)
            n77 = And(x=w389, y=w378) -> (x .and. y?=w345:bool)
            n78 = call "SIM BDF Change Order.vi"("BDF data"=w387, "Current Order"=w349, "proposed new order"=w379, "Step Accepted?"=w345) -> ("BDF data out"=w392:T15)  [unwired: 3 out]
            n79 = case shown="True" w345 {
              tunnel: w393 -> [w408 _]
              tunnel: w392 -> [w407 w416]
              tunnel: [w406 w416] -> w391
              tunnel: w358 -> [_ w424]
              tunnel: w377 -> [_ w423]
              tunnel: [w405 w422] -> w365
              tunnel: w376 -> [w405 w421]
              tunnel: [w398 w415] -> w375
              tunnel: [w397 SIM_diagram_eval_stage."Major Substep" ("Diag Eval Stage")] -> w374
              tunnel: [w396 TRUE ("Discrete step?")] -> w373
              tunnel: [w404 w417] -> w372
              tunnel: [w403 w418] -> w371
              tunnel: w370 -> [w402 w417]
              tunnel: w369 -> [w401 w418]
              tunnel: w359 -> [w400 _]
              tunnel: w361 -> [w399 _]
              tunnel: w368 -> [w398 _]
              tunnel: w367 -> [w397 _]
              tunnel: w366 -> [w396 _]
              tunnel: w354 -> [_ w412]
              tunnel: w350 -> [_ w411]
              tunnel: [_ w414] -> w353
              tunnel: w352 -> [_ w413]
              tunnel: w349 -> [_ w415]
              tunnel: w348 -> [_ w410]
              tunnel: w347 -> [_ w409]
              frame False {
                # "restore BDFs \nif step failed..."
                n80 = Bundle By Name(cluster=w407, "BDFs"=w408) -> (w406:T15)
                n81 = call "SIM Let ZC Adjust Proposed StepSize.vi"("current timestep base"=w399, "proposed step time"=w400, "proposed step size"=w401, "max step ratio"=w402) -> ("proposed step size out"=w403:dbl, "max step ratio out"=w404:dbl)  [unwired: 2 out]
              }
              frame True {
                (unwired) TRUE
                n82 = case shown="True" w424 {
                  tunnel: w423 -> [_ w426]
                  tunnel: [w425 w426] -> w422
                  tunnel: w421 -> [w425 _]
                  frame False {
                  }
                  frame True {
                  }
                }
                n83 = call "SIM Is Discrete Tick.vi"("min step size"=w409, "initial time"=w410, "time (ticks)"=w411, "tick period (sec)"=w412, "simulation time"=w413) -> ("Discrete Tick?"=w414:bool)  [unwired: 6 out]
              }
            }
            n84 = Bundle By Name(cluster=w391, "BDF stage"=SIM_BDF_stages."Choose StepSize") -> (w390:T15)
          }
          frame "Choose StepSize" {
            n85 = case shown="True" w435 {
              tunnel: w443 -> [_ w480]
              tunnel: w434 -> [w474 w479]
              tunnel: w453 -> [w473 w478]
              tunnel: [w474 w477] -> w442
              tunnel: [w473 w476] -> w452
              tunnel: [w472 TRUE ("step complete?")] -> w450
              tunnel: w451 -> [w472 _]
              frame False {
              }
              frame True {
                n86 = call "SIM update timestep base.vi"("Timestep Index"=w478, "current timestep base"=w479, "step size"=w480) -> ("Timestep Index out"=w476:dbl, "current timestep base out"=w477:dbl)  [unwired: 3 out]
              }
            }
            n87 = And(x=w432, y=w435) -> (x .and. y?=w428:bool)
            n88 = call "SIM limit new stepsize.vi"("min step size"=w447, "current timestep base"=w442, "error"=w448, "proposed step time"=w433, "proposed step size"=w449, "step size"=w443) -> ("error out"=w445:errorcluster, "proposed step size"=w446:dbl, "step size"=w444:dbl)  [unwired: 3 out]
            n89 = Not Equal?(x=w444, y=w443) -> (x != y?=w458:bool)
            n90 = case shown="True" w428 {
              tunnel: w457 -> [w464 w470]
              tunnel: [w460 w470] -> w456
              tunnel: w443 -> [w463 _]
              tunnel: w444 -> [w462 _]
              tunnel: w458 -> [w461 _]
              tunnel: [SIM_BDF_stages."Initial Guess" ("BDF stage") SIM_BDF_stages."Reset BDFs" ("BDF stage")] -> w454
              frame False {
                # "Do not exit the\nmanager - as \nlong as BDFs\nare up-to-date\nwe can go to\ninitial guess"
                n91 = case shown="True" w461 {
                  tunnel: w464 -> [w465 w469]
                  tunnel: [w465 w468] -> w460
                  tunnel: w463 -> [_ w467]
                  tunnel: w462 -> [_ w466]
                  frame False {
                  }
                  frame True {
                    n92 = call "SIM BDF resample BDs.vi"("BDF data"=w469, "current stepSize"=w467, "new stepSize"=w466) -> ("BDF data out"=w468:T15)  [unwired: 2 out]
                  }
                }
              }
              frame True {
                # "Do not exit the manager.\nProceed to reset BDFs"
              }
            }
            n93 = Bundle By Name(cluster=w456, "BDF stage"=w454) -> (w455:T15)
          }
          frame "Reset BDFs" {
            w502 = 1 ("Current Order")
            # "Do not leave the\nmanager - go on\nto initial guess"
            n94 = Unbundle By Name(w499) -> ("BDFs"=w507:dbl[][])
            n95 = Multiply(x=w497, y=w487) -> (x*y=w506:dbl[])
            n96 = Replace Array Subset(array=w507, new element #1=w498, index (row) #1=0 ("index (row)"), new element #2=w506, index (row) #2=1 ("index (row)")) -> (w503:dbl[][])  [unwired: 2 in]
            n97 = Bundle By Name(cluster=w499, "BDFs"=w503, "Current Order"=w502, "Max Err Order"=w502, "Steps This Order"=0, "reinit Jac."=TRUE) -> (w511:T15)
            n98 = Bundle By Name(cluster=w511, "BDF stage"=SIM_BDF_stages."Initial Guess") -> (w508:T15)
          }
        }
        n99 = Unbundle By Name(w25) -> ("status"=w71:bool)
        n100 = case shown="True" w68 {
          tunnel: w24 -> [w78 w85]
          tunnel: [w78 w84] -> w23
          tunnel: [w77 w83] -> w22
          tunnel: w21 -> [w77 w82]
          tunnel: w20 -> [_ w81]
          tunnel: w19 -> [_ w80]
          tunnel: w18 -> [_ w79]
          frame False {
          }
          frame True {
            n101 = call "SIM limit signal (array).vi"("lower limits"=w80, "upper limits"=w81, "limit types"=w79, "limited? in"=w82, "inputs"=w85) -> ("limited? out"=w83:bool[], "outputs"=w84:dbl[])  [unwired: 1 in, 4 out]
          }
        }
        n102 = Or(x=w71, y=w68) -> (x .or. y?=w74:bool)
        n103 = Not Equal?(x=w12, y=SIM_diagram_eval_stage."Major Substep") -> (x != y?=w13:bool)
        n104 = Select(t=w9, s=w13, f=w10) -> (s? t:f=w8:dbl)
        n105 = Bundle By Name(cluster=w17, "Simulation Registry.Cont State data.outputs"=w23, "Simulation Registry.Cont State data.inputs"=w39, "Simulation Registry.Cont State data.limited?"=w22, "Diag Eval Stage"=w12, "Substep Index"=w65, "simulation time"=w63, "Discrete step?"=w61, "Simulation Registry.DiscreteInfo.discrete \ntick?"=w59, "current timestep base"=w57, "step accepted?"=w55, "step complete?"=w53, "proposed step time"=w8, "reset integrator?"=w50, "step size"=w48, "proposed step size"=w46, "Timestep Index"=w44, "max step ratio"=w42, "error"=w25, "Method Order"=w28) -> (w37:T1)
      }
    }
    frame True {
      w514 = TRUE ("step accepted?")
      n106 = Bundle By Name(cluster=w512, "step accepted?"=w514, "step complete?"=w514) -> (w513:T1)
    }
  }
  "Simulation data out" <- w5
